vi "DAQ_Status_Read.vi"(1 "channel":T1) -> (0 "state":string)   [LabVIEW 2024]
uses:
  <extravilib>/ChannelInstances/Stream-str/)Channel.ctl
  <extravilib>/ChannelInstances/Stream-str/Read With Abort.vi
  <extravilib>/ChannelInstances/Stream-str/EndpointRead.vi
  <extravilib>/ChannelInstances/Stream-str/)Channel.vi
  <resource>/ChannelSupport/_ChannelSupport/WaitIfNeeded.vi
  <extravilib>/ChannelInstances/Stream-str.lvlib
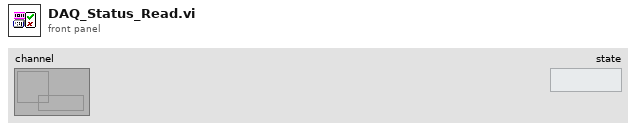
[diagram p1: front panel]
types:
  T1 = typedef "Stream-str.lvlib/)Channel.ctl" = refnum<queue>
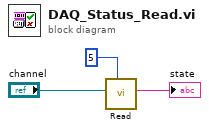
[diagram p0: block diagram]
diagram:
  n1 = call <extravilib>:"Read.vi"("timeout in ms (-1)"=5, "channel"="channel") -> ("element"=→"state":string)  [unwired: 5 in, 4 out]
